vi "HDF5_Init_Weather_Refs.vi"(8 "error in":errorcluster, 9 "File Exists?":bool, 10 "HDF5 file ref 2":T1 format="%.0x") -> (0 "error out":errorcluster, 2 "HDF5 file ref":T1 format="%.0x", 3 "Weath_Refs":T2 {"WindDirSTD_dset" format="%.0x"; "WindGusts_dset" format="%.0x"; "RainFall_dset" format="%.0x"; "RainRate_dset" format="%.0x"; "Pressure_dset" format="%.0x"; "Humidity_dset" format="%.0x"; "Temp_dset" format="%.0x"; "WindDir_dset" format="%.0x"; "WindSpd_dset" format="%.0x"; "TimeStamp_dset" format="%.0x"; "Group_ref" format="%.0x"; "TimeString_dset" format="%.0x"})   [LabVIEW 2018]
uses:
  <vilib>/addons/h5labview2/base/hid_t.ctl
  Controls/Clusts/WeatherRefs.ctl
  lib_path_mod_20200519.vi
  <vilib>/addons/h5labview2/base/H5Equery.vi
  <vilib>/addons/h5labview2/attrib/H5Awrite.llb/H5Awrite.xnode
  <vilib>/addons/h5labview2/group/H5G.lvlib
  <vilib>/addons/h5labview2/dataset/H5D.lvlib
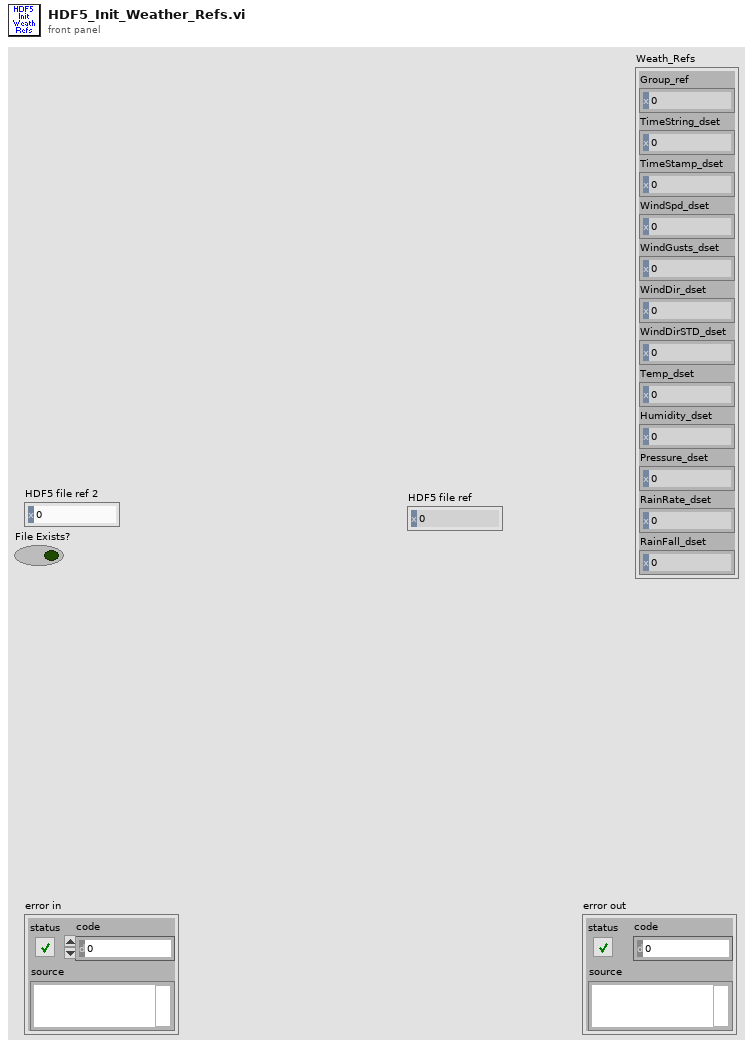
[diagram p1: front panel]
types:
  T1 = typedef "hid_t.ctl" = i32
  T2 = typedef "WeatherRefs.ctl" = cluster{"Group_ref":T1, "TimeString_dset":T1, "TimeStamp_dset ":T1, "WindSpd_dset":T1, "WindGusts_dset":T1, "WindDir_dset":T1, "WindDirSTD_dset":T1, "Temp_dset":T1, "Humidity_dset":T1, "Pressure_dset":T1, "RainRate_dset":T1, "RainFall_dset":T1}
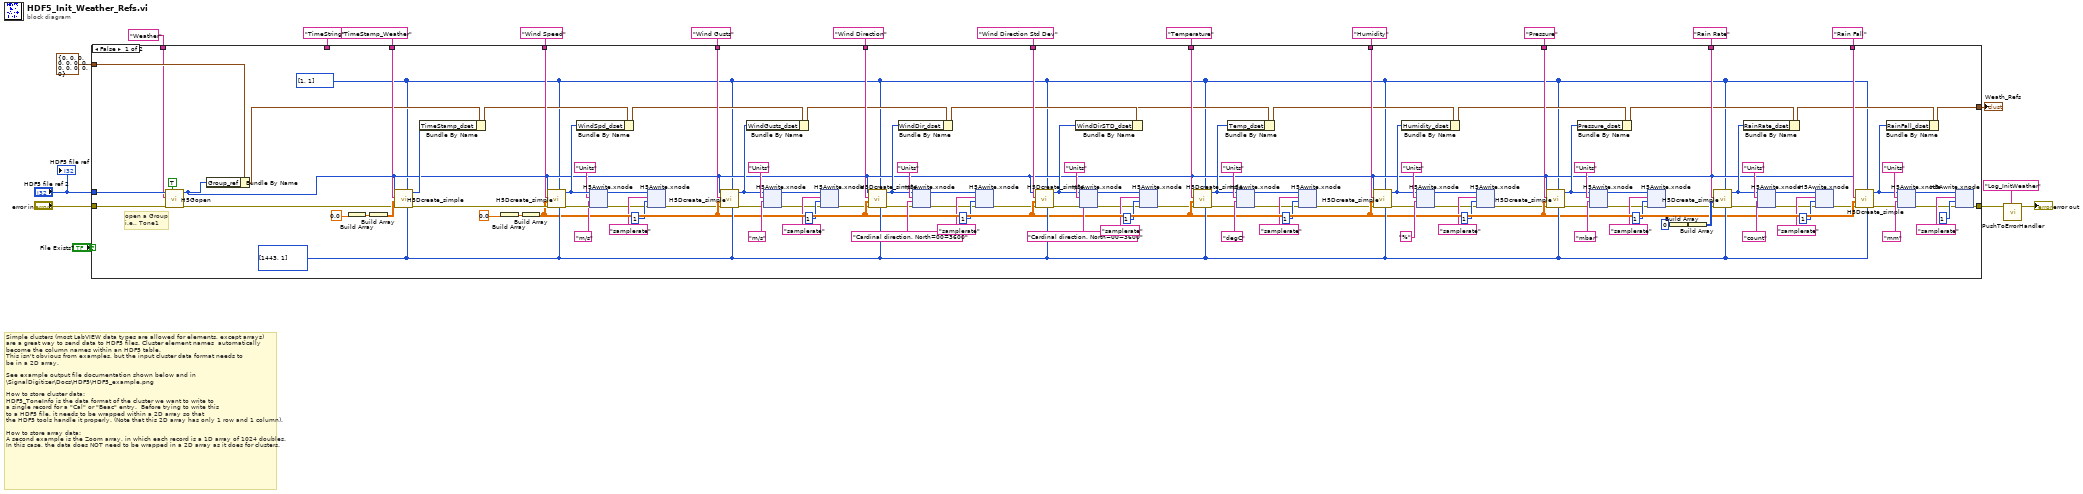
[diagram p0: block diagram]
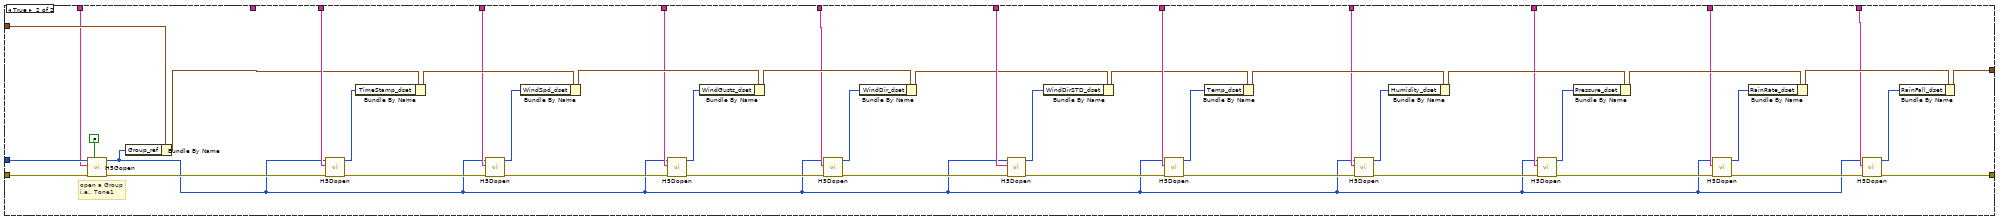
[diagram p2: hidden frame]
diagram:
  # "Simple clusters (most LabVIEW data types are allowed for elements, except arrays) \nare a great way to send data to HDF5 files. Cluster element names  automatically\nbecome the column names within an HDF5 table.\nThis isn't obvious from examples, but the input cluster data format needs to \nbe in a 2D array.\n\nSee example output file documentation shown below and in\n\\SignalDigitizer\\Docs\\HDF5\\HDF5_example.png\n\nHow to store cluster data:\nHDF5_ToneInfo is the data format of the cluster we want to write to \na single record for a \"Cal\" or \"Beac\" entry.  Before trying to write this \nto a HDF5 file, it needs to be wrapped within a 2D array so that \nthe HDF5 tools handle it properly. (Note that this 2D array has only 1 row and 1 column).\n\nHow to store array data:\nA second example is the Zoom array, in which each record is a 1D array of 1024 doubles.\nIn this case, the data does NOT need to be wrapped in a 2D array as it does for clusters."
  n1 = case shown="False" "File Exists?" {
    tunnel: "error in" -> [w142 w532]
    tunnel: "HDF5 file ref 2" -> [w141 w531]
    tunnel: [w21 w494] -> w3
    tunnel: T2 {"Group_ref"=0, "TimeString_dset"=0, "TimeStamp_dset "=0, "WindSpd_dset"=0, "WindGusts_dset"=0, "WindDir_dset"=0, "WindDirSTD_dset"=0, "Temp_dset"=0, "Humidity_dset"=0, "Pressure_dset"=0, "RainRate_dset"=0, "RainFall_dset"=0} ("Cluster") -> [w139 w529]
    tunnel: [w122 w511] -> w16
    tunnel: "TimeString" ("string") -> [_ _]
    tunnel: "Weather" ("name") -> [w138 w528]
    tunnel: "TimeStamp_Weather" ("string") -> [w131 w510]
    tunnel: "Wind Speed" ("string") -> [w130 w509]
    tunnel: "Wind Gusts" ("string") -> [w129 w508]
    tunnel: "Wind Direction" ("string") -> [w128 w507]
    tunnel: "Temperature" ("string") -> [w127 w506]
    tunnel: "Humidity" ("string") -> [w126 w505]
    tunnel: "Pressure" ("string") -> [w125 w504]
    tunnel: "Rain Rate" ("string") -> [w124 w503]
    tunnel: "Rain Fall" ("string") -> [w123 w502]
    tunnel: "Wind Direction Std Dev" ("string") -> [w74 w491]
    frame False {
      w66 = i32[] [1, 1] ("size(s)")
      w75 = u64[] [1443, 1] ("max size")
      # "open a Group\ni.e., Tone1"
      n2 = call <vilib>:"H5Gopen.vi"("create? (F)"=TRUE, "error in (no error)"=w142, "name"=w138, "ref in"=w141) -> ("error out"=w69:errorcluster, "group out"=w67:T1)  [unwired: 6 in]
      n3 = Bundle By Name(cluster=w139, "Group_ref"=w67) -> (w68:T2)
      n4 = Build Array(0.0 ("Timestamp")) -> (w136:dbl[])
      n5 = Build Array(w136) -> (w137:dbl[][])
      n6 = call <vilib>:"H5Dcreate_simple.vi"("max size"=w75, "chunk size"=w66, "error in (no error)"=w69, "type in"=w137, "name"=w131, "ref in"=w67) -> ("error out"=w111:errorcluster, "dset out"=w135:T1)  [unwired: 4 in]
      n7 = Bundle By Name(cluster=w68, "TimeStamp_dset"=w135) -> (w115:T2)
      n8 = Build Array(sgl 0.0 ("Wind Speed")) -> (w134:sgl[])
      n9 = Build Array(w134) -> (w70:sgl[][])
      n10 = call <vilib>:"H5Dcreate_simple.vi"("max size"=w75, "chunk size"=w66, "error in (no error)"=w111, "type in"=w70, "name"=w130, "ref in"=w67) -> ("error out"=w110:errorcluster, "dset out"=w109:T1)  [unwired: 4 in]
      n11 = Bundle By Name(cluster=w115, "WindSpd_dset"=w109) -> (w116:T2)
      n12 = xnode "H5Awrite.xnode"("error in (no error)"=w110, "data"="m/s" ("Name"), "attrib name"="Units", "ref in"=w109) -> ("error out"=w62:errorcluster, "ref out"=w63:i32)  [unwired: 3 in, 1 out]
      n13 = xnode "H5Awrite.xnode"("error in (no error)"=w62, "data"=u32 1, "attrib name"="samplerate", "ref in"=w63) -> ("error out"=w61:errorcluster)  [unwired: 3 in, 2 out]
      n14 = call <vilib>:"H5Dcreate_simple.vi"("max size"=w75, "chunk size"=w66, "error in (no error)"=w61, "type in"=w70, "name"=w129, "ref in"=w67) -> ("error out"=w92:errorcluster, "dset out"=w91:T1)  [unwired: 4 in]
      n15 = Bundle By Name(cluster=w116, "WindGusts_dset"=w91) -> (w117:T2)
      n16 = xnode "H5Awrite.xnode"("error in (no error)"=w92, "data"="m/s" ("Name"), "attrib name"="Units", "ref in"=w91) -> ("error out"=w57:errorcluster, "ref out"=w58:i32)  [unwired: 3 in, 1 out]
      n17 = xnode "H5Awrite.xnode"("error in (no error)"=w57, "data"=u32 1, "attrib name"="samplerate", "ref in"=w58) -> ("error out"=w56:errorcluster)  [unwired: 3 in, 2 out]
      n18 = call <vilib>:"H5Dcreate_simple.vi"("max size"=w75, "chunk size"=w66, "error in (no error)"=w56, "type in"=w70, "name"=w128, "ref in"=w67) -> ("error out"=w89:errorcluster, "dset out"=w90:T1)  [unwired: 4 in]
      n19 = Bundle By Name(cluster=w117, "WindDir_dset"=w90) -> (w73:T2)
      n20 = xnode "H5Awrite.xnode"("error in (no error)"=w89, "data"="Cardinal direction, North=00=3600" ("Name"), "attrib name"="Units", "ref in"=w90) -> ("error out"=w52:errorcluster, "ref out"=w53:i32)  [unwired: 3 in, 1 out]
      n21 = xnode "H5Awrite.xnode"("error in (no error)"=w52, "data"=u32 1, "attrib name"="samplerate", "ref in"=w53) -> ("error out"=w51:errorcluster)  [unwired: 3 in, 2 out]
      n22 = call <vilib>:"H5Dcreate_simple.vi"("max size"=w75, "chunk size"=w66, "error in (no error)"=w51, "type in"=w70, "name"=w74, "ref in"=w67) -> ("error out"=w78:errorcluster, "dset out"=w71:T1)  [unwired: 4 in]
      n23 = Bundle By Name(cluster=w73, "WindDirSTD_dset"=w71) -> (w72:T2)
      n24 = xnode "H5Awrite.xnode"("error in (no error)"=w78, "data"="Cardinal direction, North=00=3600" ("Name"), "attrib name"="Units", "ref in"=w71) -> ("error out"=w47:errorcluster, "ref out"=w48:i32)  [unwired: 3 in, 1 out]
      n25 = xnode "H5Awrite.xnode"("error in (no error)"=w47, "data"=u32 1, "attrib name"="samplerate", "ref in"=w48) -> ("error out"=w46:errorcluster)  [unwired: 3 in, 2 out]
      n26 = call <vilib>:"H5Dcreate_simple.vi"("max size"=w75, "chunk size"=w66, "error in (no error)"=w46, "type in"=w70, "name"=w127, "ref in"=w67) -> ("error out"=w88:errorcluster, "dset out"=w79:T1)  [unwired: 4 in]
      n27 = Bundle By Name(cluster=w72, "Temp_dset"=w79) -> (w118:T2)
      n28 = xnode "H5Awrite.xnode"("error in (no error)"=w88, "data"="degC" ("Name"), "attrib name"="Units", "ref in"=w79) -> ("error out"=w42:errorcluster, "ref out"=w43:i32)  [unwired: 3 in, 1 out]
      n29 = xnode "H5Awrite.xnode"("error in (no error)"=w42, "data"=u32 1, "attrib name"="samplerate", "ref in"=w43) -> ("error out"=w41:errorcluster)  [unwired: 3 in, 2 out]
      n30 = call <vilib>:"H5Dcreate_simple.vi"("max size"=w75, "chunk size"=w66, "error in (no error)"=w41, "type in"=w70, "name"=w126, "ref in"=w67) -> ("error out"=w87:errorcluster, "dset out"=w80:T1)  [unwired: 4 in]
      n31 = Bundle By Name(cluster=w118, "Humidity_dset"=w80) -> (w119:T2)
      n32 = xnode "H5Awrite.xnode"("error in (no error)"=w87, "data"="%" ("Name"), "attrib name"="Units", "ref in"=w80) -> ("error out"=w37:errorcluster, "ref out"=w38:i32)  [unwired: 3 in, 1 out]
      n33 = xnode "H5Awrite.xnode"("error in (no error)"=w37, "data"=u32 1, "attrib name"="samplerate", "ref in"=w38) -> ("error out"=w36:errorcluster)  [unwired: 3 in, 2 out]
      n34 = call <vilib>:"H5Dcreate_simple.vi"("max size"=w75, "chunk size"=w66, "error in (no error)"=w36, "type in"=w70, "name"=w125, "ref in"=w67) -> ("error out"=w86:errorcluster, "dset out"=w81:T1)  [unwired: 4 in]
      n35 = Bundle By Name(cluster=w119, "Pressure_dset"=w81) -> (w120:T2)
      n36 = xnode "H5Awrite.xnode"("error in (no error)"=w86, "data"="mbar" ("Name"), "attrib name"="Units", "ref in"=w81) -> ("error out"=w33:errorcluster, "ref out"=w32:i32)  [unwired: 3 in, 1 out]
      n37 = xnode "H5Awrite.xnode"("error in (no error)"=w33, "data"=u32 1, "attrib name"="samplerate", "ref in"=w32) -> ("error out"=w31:errorcluster)  [unwired: 3 in, 2 out]
      n38 = Build Array(i16 0 ("Rain Rate")) -> (w133:i16[])
      n39 = Build Array(w133) -> (w132:i16[][])
      n40 = call <vilib>:"H5Dcreate_simple.vi"("max size"=w75, "chunk size"=w66, "error in (no error)"=w31, "type in"=w132, "name"=w124, "ref in"=w67) -> ("error out"=w85:errorcluster, "dset out"=w82:T1)  [unwired: 4 in]
      n41 = Bundle By Name(cluster=w120, "RainRate_dset"=w82) -> (w121:T2)
      n42 = xnode "H5Awrite.xnode"("error in (no error)"=w85, "data"="count" ("Name"), "attrib name"="Units", "ref in"=w82) -> ("error out"=w28:errorcluster, "ref out"=w27:i32)  [unwired: 3 in, 1 out]
      n43 = xnode "H5Awrite.xnode"("error in (no error)"=w28, "data"=u32 1, "attrib name"="samplerate", "ref in"=w27) -> ("error out"=w26:errorcluster)  [unwired: 3 in, 2 out]
      n44 = call <vilib>:"H5Dcreate_simple.vi"("max size"=w75, "chunk size"=w66, "error in (no error)"=w26, "type in"=w70, "name"=w123, "ref in"=w67) -> ("error out"=w84:errorcluster, "dset out"=w83:T1)  [unwired: 4 in]
      n45 = Bundle By Name(cluster=w121, "RainFall_dset"=w83) -> (w122:T2)
      n46 = xnode "H5Awrite.xnode"("error in (no error)"=w84, "data"="mm" ("Name"), "attrib name"="Units", "ref in"=w83) -> ("error out"=w23:errorcluster, "ref out"=w22:i32)  [unwired: 3 in, 1 out]
      n47 = xnode "H5Awrite.xnode"("error in (no error)"=w23, "data"=u32 1, "attrib name"="samplerate", "ref in"=w22) -> ("error out"=w21:errorcluster)  [unwired: 3 in, 2 out]
    }
    frame True {
      # "open a Group\ni.e., Tone1"
      n48 = call <vilib>:"H5Gopen.vi"("create? (F)"=FALSE, "error in (no error)"=w532, "name"=w528, "ref in"=w531) -> ("error out"=w492:errorcluster, "group out"=w485:T1)  [unwired: 6 in]
      n49 = Bundle By Name(cluster=w529, "Group_ref"=w485) -> (w493:T2)
      n50 = call <vilib>:"H5Dopen.vi"("error in (no error)"=w492, "name"=w510, "loc in"=w485) -> ("error out"=w501:errorcluster, "dset out"=w527:T1)  [unwired: 7 in]
      n51 = Bundle By Name(cluster=w493, "TimeStamp_dset"=w527) -> (w518:T2)
      n52 = call <vilib>:"H5Dopen.vi"("error in (no error)"=w501, "name"=w509, "loc in"=w485) -> ("error out"=w500:errorcluster, "dset out"=w526:T1)  [unwired: 7 in]
      n53 = Bundle By Name(cluster=w518, "WindSpd_dset"=w526) -> (w517:T2)
      n54 = call <vilib>:"H5Dopen.vi"("error in (no error)"=w500, "name"=w508, "loc in"=w485) -> ("error out"=w499:errorcluster, "dset out"=w525:T1)  [unwired: 7 in]
      n55 = Bundle By Name(cluster=w517, "WindGusts_dset"=w525) -> (w516:T2)
      n56 = call <vilib>:"H5Dopen.vi"("error in (no error)"=w499, "name"=w507, "loc in"=w485) -> ("error out"=w490:errorcluster, "dset out"=w524:T1)  [unwired: 7 in]
      n57 = Bundle By Name(cluster=w516, "WindDir_dset"=w524) -> (w488:T2)
      n58 = call <vilib>:"H5Dopen.vi"("error in (no error)"=w490, "name"=w491, "loc in"=w485) -> ("error out"=w489:errorcluster, "dset out"=w486:T1)  [unwired: 7 in]
      n59 = Bundle By Name(cluster=w488, "WindDirSTD_dset"=w486) -> (w487:T2)
      n60 = call <vilib>:"H5Dopen.vi"("error in (no error)"=w489, "name"=w506, "loc in"=w485) -> ("error out"=w498:errorcluster, "dset out"=w523:T1)  [unwired: 7 in]
      n61 = Bundle By Name(cluster=w487, "Temp_dset"=w523) -> (w515:T2)
      n62 = call <vilib>:"H5Dopen.vi"("error in (no error)"=w498, "name"=w505, "loc in"=w485) -> ("error out"=w497:errorcluster, "dset out"=w522:T1)  [unwired: 7 in]
      n63 = Bundle By Name(cluster=w515, "Humidity_dset"=w522) -> (w514:T2)
      n64 = call <vilib>:"H5Dopen.vi"("error in (no error)"=w497, "name"=w504, "loc in"=w485) -> ("error out"=w496:errorcluster, "dset out"=w521:T1)  [unwired: 7 in]
      n65 = Bundle By Name(cluster=w514, "Pressure_dset"=w521) -> (w513:T2)
      n66 = call <vilib>:"H5Dopen.vi"("error in (no error)"=w496, "name"=w503, "loc in"=w485) -> ("error out"=w495:errorcluster, "dset out"=w520:T1)  [unwired: 7 in]
      n67 = Bundle By Name(cluster=w513, "RainRate_dset"=w520) -> (w512:T2)
      n68 = call <vilib>:"H5Dopen.vi"("error in (no error)"=w495, "name"=w502, "loc in"=w485) -> ("error out"=w494:errorcluster, "dset out"=w519:T1)  [unwired: 7 in]
      n69 = Bundle By Name(cluster=w512, "RainFall_dset"=w519) -> (w511:T2)
    }
  }
  "Weath_Refs" <- w16
  n70 = call "PushToErrorHandler.vi"("ErrorIn"=w3, "ErrorLocation"="Log_InitWeather") -> ("ErrorOut"=→"error out":errorcluster)  [unwired: 5 in]
  "HDF5 file ref" <- "HDF5 file ref 2"
